vi "开始界面.vi"() -> ()   [LabVIEW 2018]
panel:
  in  "VI路径":path=path "D:/Labviewprogram/登录界面/主界面.vi"
  in  "密码文件":path=path "D:/Labviewprogram/登录界面/密码.txt"
  in  "账户文件":path=path "D:/Labviewprogram/登录界面/账户.txt"
  out "登录按钮":bool
  in  "密   码":string
  in  "用户名":string
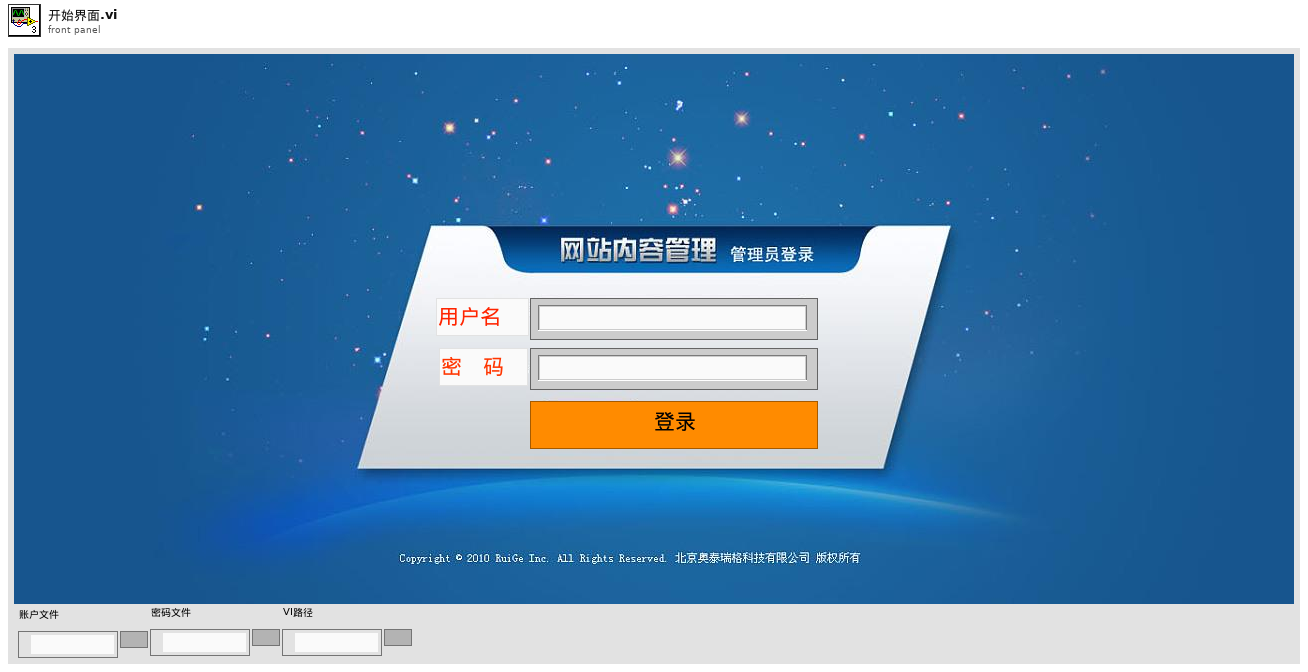
[diagram p1: front panel]
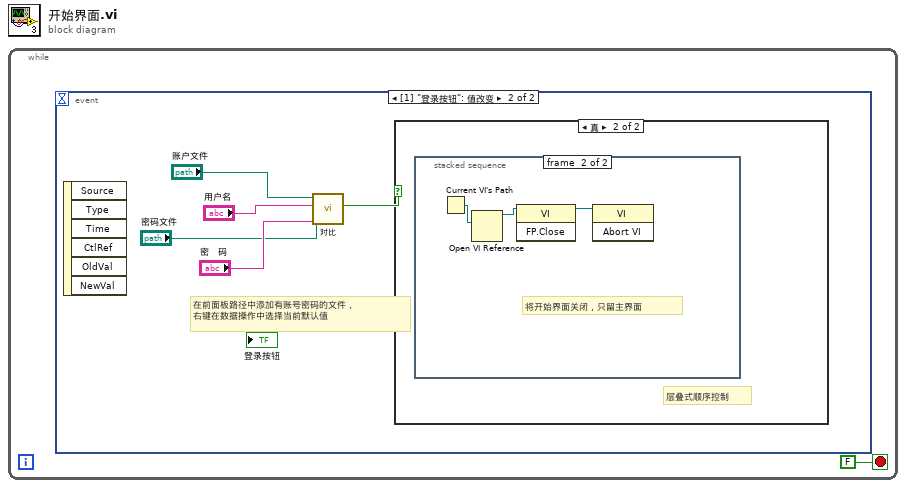
[diagram p0: block diagram]
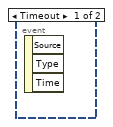
[diagram p2: hidden frame]
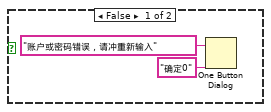
[diagram p3: hidden frame]
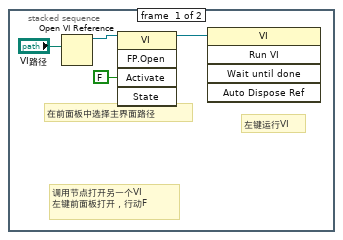
[diagram p4: hidden frame]
diagram:
  n1 = while {
    stop <- FALSE stop-if-true
    n2 = event shown="[1] \"登录按钮\": 值改变" {
      selector: _ -> [_ _]
      dyn-events: _ -> [_ _]
      timeout: _ -> [_ _]
      event Timeout {
        n3 = event-data() -> ()  [unwired: 1 in, 3 out]
      }
      event "登录按钮": Value Change {
        # "在前面板路径中添加有账号密码的文件，\n右键在数据操作中选择当前默认值"
        n4 = event-data() -> ()  [unwired: 1 in, 6 out]
        n5 = call "对比.vi"("密码"="密   码", "密码文件"="密码文件", "账户"="用户名", "账户文件"="账户文件") -> ("x与y？"=w2:bool)  [unwired: 7 in]
        n6 = case shown="真" w2 {
          frame False {
            n7 = One Button Dialog(message="账户或密码错误，请冲重新输入" ("消息"), button name ("OK")="确定0" ("按钮名称（“确定”）")) -> ()  [unwired: 1 out]
          }
          frame True {
            # "层叠式顺序控制"
            n8 = stacked-sequence {
              frame #0 {
                # "在前面板中选择主界面路径"
                # "左键运行VI"
                # "调用节点打开另一个VI\n左键前面板打开，行动F"
                n9 = Open VI Reference(vi path="VI路径") -> (vi reference=w12:refnum<vi>)  [unwired: 5 in, 1 out]
                n10 = invoke class="VI" method="FP.Open"(reference=w12, "Activate"=FALSE ("激活？")) -> (reference out=w10:refnum<vi>)  [unwired: 3 in, 4 out]
                n11 = invoke class="VI" method="Run VI"(reference=w10) -> ()  [unwired: 4 in, 5 out]
              }
              frame #1 {
                # "将开始界面关闭，只留主界面"
                n12 = Current VI's Path() -> (path=w15:path)
                n13 = Open VI Reference(vi path=w15) -> (vi reference=w14:refnum<vi>)  [unwired: 5 in, 1 out]
                n14 = invoke class="VI" method="FP.Close"(reference=w14) -> (reference out=w13:refnum<vi>)  [unwired: 2 in, 2 out]
                n15 = invoke class="VI" method="Abort VI"(reference=w13) -> ()  [unwired: 2 in, 3 out]
              }
            }
          }
        }
      }
    }
  }
